vi "Stamp From Iteration.vi"(9 "Rate (Hz)":dbl format="%#_13g", 10 "frame_id":string, 11 "Iteration":i32) -> (3 "Header":T1)   [LabVIEW 2013, in "Helpers.lvlib"]
uses:
  Helpers.lvlib
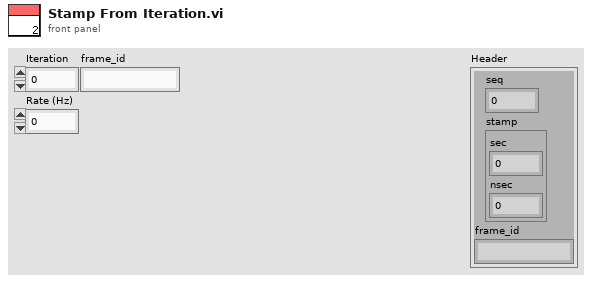
[diagram p1: front panel]
types:
  T1 = cluster{"seq":u32, "stamp":cluster{"sec":i32, "nsec":i32}, "frame_id":string}
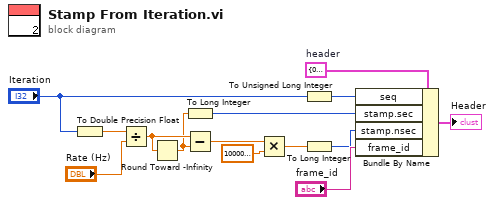
[diagram p0: block diagram]
diagram:
  w12 = T1 {"seq"=0, "stamp"={"sec"=0, "nsec"=0}, "frame_id"=""}  # header
  n1 = To Double Precision Float(number="Iteration") -> (double precision float=w14:dbl)
  n2 = Divide(x=w14, y="Rate (Hz)") -> (x/y=w7:dbl)
  n3 = Round Toward -Infinity(1:w7) -> (0:w6:dbl)
  n4 = To Long Integer(number=w6) -> (32bit integer=w8:i32)
  n5 = Subtract(x=w7, y=w6) -> (x-y=w5:dbl)
  n6 = Multiply(x=w5, y=1000000000.0) -> (x*y=w3:dbl)
  n7 = To Unsigned Long Integer(number="Iteration") -> (unsigned 32bit integer=w10:u32)
  n8 = To Long Integer(number=w3) -> (32bit integer=w2:i32)
  n9 = Bundle By Name(cluster=w12, "seq"=w10, "stamp.sec"=w8, "stamp.nsec"=w2, "frame_id"="frame_id") -> (→"Header":T1)
